vi "Timer Thing.vi"() -> (3 "Time has Elapsed":bool)   [LabVIEW 2013]
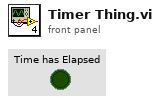
[diagram p1: front panel]
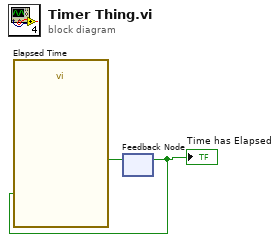
[diagram p0: block diagram]
diagram:
  n1 = feedback #1() -> (w1:bool)  [unwired: 1 in]
  "Time has Elapsed" <- w1
  n2 = call "Elapsed Time"("Reset"=w1) -> ("Time has Elapsed"=w2:bool)  [unwired: 11 in, 7 out]
  n3 = feedback-in #1(w2) -> ()
